vi "Write Interface.lvclass.vi"(8 "error in (no error)":errorcluster, 10 "Interface.lvclass":refnum<class "Interface.lvclass">, 11 "JSON reader in":refnum<class "JSON reader.lvclass">) -> (0 "error out":errorcluster, 3 "JSON reader out":refnum<class "JSON reader.lvclass">)   [LabVIEW 2018, in "JSON reader.lvclass"]
uses:
  JSON reader.lvclass
  Interface/Interface.lvclass
  JSON reader.lvclass/JSON reader.ctl
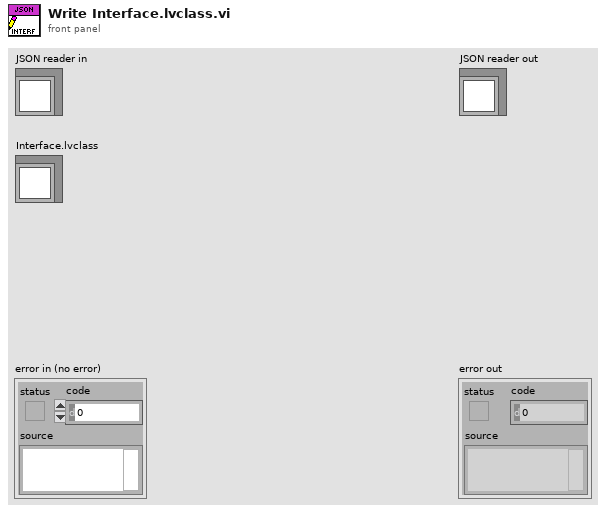
[diagram p1: front panel]
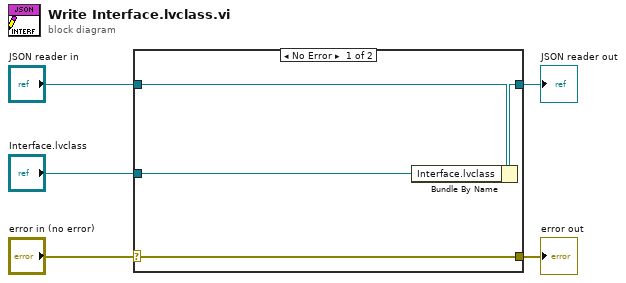
[diagram p0: block diagram]
diagram:
  n1 = case shown="No Error" "error in (no error)" {
    selector: "error in (no error)" -> [w9 w10]
    tunnel: [w9 w10] -> w4
    tunnel: [w7 w11] -> w2
    tunnel: "JSON reader in" -> [w8 w11]
    tunnel: "Interface.lvclass" -> [w6 _]
    frame No Error {
      n2 = Bundle By Name(cluster=w8, "Interface.lvclass"=w6) -> (w7:refnum<class "JSON reader.lvclass">)
    }
    frame Error {
    }
  }
  "error out" <- w4
  "JSON reader out" <- w2
